vi "Get Payload.vi"(8 "error in (no error)":errorcluster, 11 "CAN Frame in":refnum<class "CAN Frame.lvclass">) -> (0 "error out":errorcluster, 2 "Payload":u8[](array[numeric]), 3 "CAN Frame out":refnum<class "CAN Frame.lvclass">)   [LabVIEW 2023, in "CAN Frame.lvclass"]
uses:
  CAN Frame.lvclass
  CAN Frame.lvclass/CAN Frame.ctl
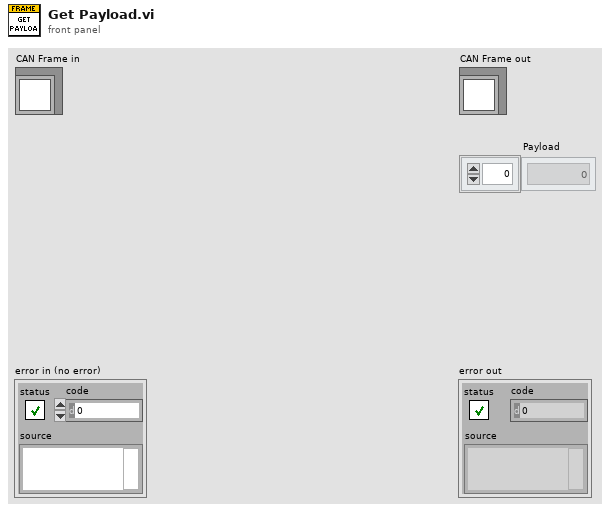
[diagram p1: front panel]
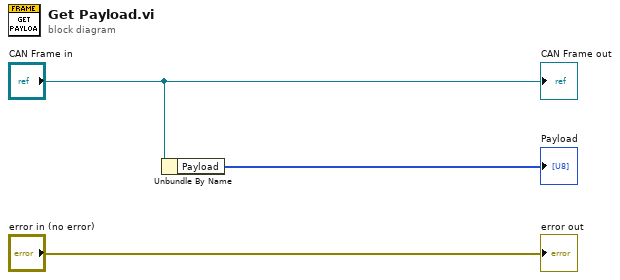
[diagram p0: block diagram]
diagram:
  n1 = Unbundle By Name("CAN Frame in") -> ("Payload"=→"Payload":u8[])
  "error out" <- "error in (no error)"
  "CAN Frame out" <- "CAN Frame in"
